vi "Teleop.vi"(10 "Match Info":T2={"Autonomous Elapsed Seconds"=0.0, "TeleOp Elapsed Seconds"=0.0, "Disabled Elapsed Seconds"=0.0, "Visited Autonomous"=FALSE, "Visited TeleOp"=FALSE, "Visited Disabled"=FALSE, "Autonomous Settings"={"Autonomous Style"=enum."Independent", "VI Refnum"=refnum}}, 11 "Call Context":T3) -> ()   [LabVIEW 2012]
doc: "This VI is called for each TeleOp packet received from the DS where the robot is not disabled. It is often used to read from the joysticks and update I/O or to update setpoints for timed control loops. It should complete and return within 20 milliseconds or it may miss DS packets."
uses:
  <vilib>/Rock Robotics/WPI/DriverStation/WPI_DriverStationDerivedRobotMode.ctl
  <vilib>/Rock Robotics/WPI/DriverStation/WPI_DriverStationMatch Info.ctl
  <vilib>/Rock Robotics/WPI/Relay/WPI_RelayValue.ctl
  Robot Global Data.vi
  <vilib>/Rock Robotics/WPI/Joystick/WPI_JoystickGetSetRefNum.vi
panel:
  in  "Roller Speed":dbl=0.75
  in  "RelayValue 2":T1
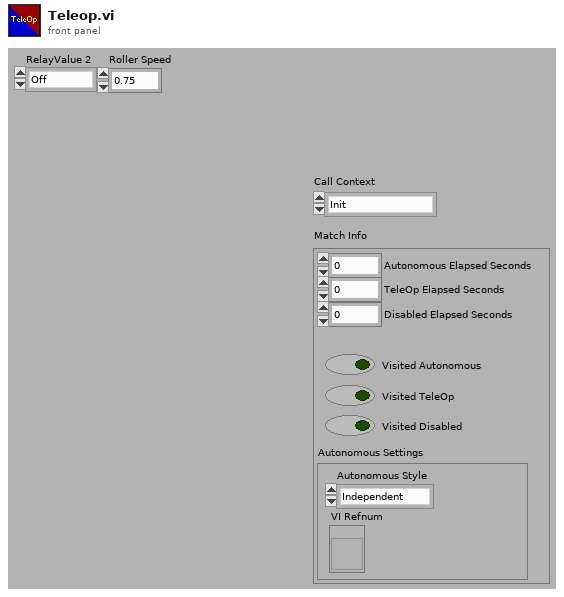
[diagram p1: front panel]
types:
  T1 = typedef "WPI_RelayValue.ctl" = enum16{"Off", "On", "Forward", "Reverse"}
  T2 = typedef "WPI_DriverStationMatch Info.ctl" = cluster{"Autonomous Elapsed Seconds":dbl, "TeleOp Elapsed Seconds":dbl, "Disabled Elapsed Seconds":dbl, "Visited Autonomous":bool, "Visited TeleOp":bool, "Visited Disabled":bool, "Autonomous Settings":cluster{"Autonomous Style":enum16{"Iterative", "Independent"}, "VI Refnum":refnum<vi>}}
  T3 = typedef "WPI_DriverStationDerivedRobotMode.ctl" = enum16{"Init", "Execute", "Stop"}
  T4 = typedef "WPI_ServoDeviceRef.ctl" = cluster{"DeviceStatus":errorcluster, "Digital Module":T5, "PWM Channel":T6, "DeadBand":T7}
  T5 = typedef "FPGA_TypedefDigitalModule.ctl" = enum16{"Digital Module 1", "Digital Module 2"}
  T6 = typedef "FPGA_DIOPWMChannel.ctl" = enum8{"PWM 1", "PWM 2", "PWM 3", "PWM 4", "PWM 5", "PWM 6", "PWM 7", "PWM 8", "PWM 9", "PWM 10", "Invalid"}
  T7 = typedef "WPI_PWMDeadband.ctl" = cluster{"Name":string, "maxPositivePwm":i32, "minPositivePwm":i32, "centerPwm":i32, "maxNegativePwm":i32, "minNegativePwm":i32, "angularRange":u16}
  T8 = typedef "WPI_MotorControlDeviceRef.ctl" = cluster{"DeviceStatus":errorcluster, "Type":enum16{"PWM", "CAN"}, "PWM":cluster{"Digital Module":T5, "PWM Channel":T6, "DeadBand":T7}, "CAN":cluster{"Device Number":u8, "Control Mode":T9, "Semaphore":T10, "Max Vout":dbl}, "Invert":bool, "TransformRef":T11, "InvTransformRef":T11}
  T9 = typedef "WPI_CANJaguar_ControlMode.ctl" = enum8{"Percent VBus", "Current", "Speed", "Position", "Voltage"}
  T10 = typedef "Semaphore RefNum" = refnum<k1>
  T11 = typedef "WPI_PWMTransform_ConPane.ctl" = refnum<vi>
  T12 = typedef "WPI_RelayDevRef.ctl" = cluster{"DevStatus":errorcluster, "Relay Channel":T13, "Digital Module":T5, "Relay Direction":T14}
  T13 = typedef "FPGA_DIORelayChannel.ctl" = enum8{"Relay 1", "Relay 2", "Relay 3", "Relay 4", "Relay 5", "Relay 6", "Relay 7", "Relay 8", "Invalid"}
  T14 = typedef "WPI_RelayDirection.ctl" = enum16{"Both directions", "Forward only", "Reverse only"}
  T15 = cluster{"Driver Station Digital Input (1-8)[0]":bool, "Driver Station Digital Input (1-8)[1]":bool, "Driver Station Digital Input (1-8)[2]":bool, "Driver Station Digital Input (1-8)[3]":bool, "Driver Station Digital Input (1-8)[4]":bool, "Driver Station Digital Input (1-8)[5]":bool, "Driver Station Digital Input (1-8)[6]":bool, "Driver Station Digital Input (1-8)[7]":bool, "Driver Station Digital Input (1-8)[8]":bool}
  T16 = cluster{"Right Servo High":dbl, "Right Servo Mid":dbl, "Right Servo Low":dbl, "Left Servo High":dbl, "Left Servo Mid":dbl, "Left Servo Low":dbl}
  T17 = typedef "WPI_JoystickDevRef.ctl" = cluster{"Device":T18}
  T18 = typedef "WPI_JoystickDeviceEnum.ctl" = enum16{"USB 1", "USB 2", "USB 3", "USB 4", "Kinect 1", "Kinect 2"}
  T19 = cluster{"axis 1 (x)":dbl, "axis 2 (y)":dbl, "axis 3 (throttle)":dbl, "axis 4":dbl, "axis 5":dbl, "axis 6":dbl}
  T20 = typedef "WPI_JoystickButtonState.ctl" = cluster{"Button 1":bool, "Button 2":bool, "Button 3":bool, "Button 4":bool, "Button 5":bool, "Button 6":bool, "Button 7":bool, "Button 8":bool, "Button 9":bool, "Button 10":bool, "Button 11":bool, "Button 12":bool}
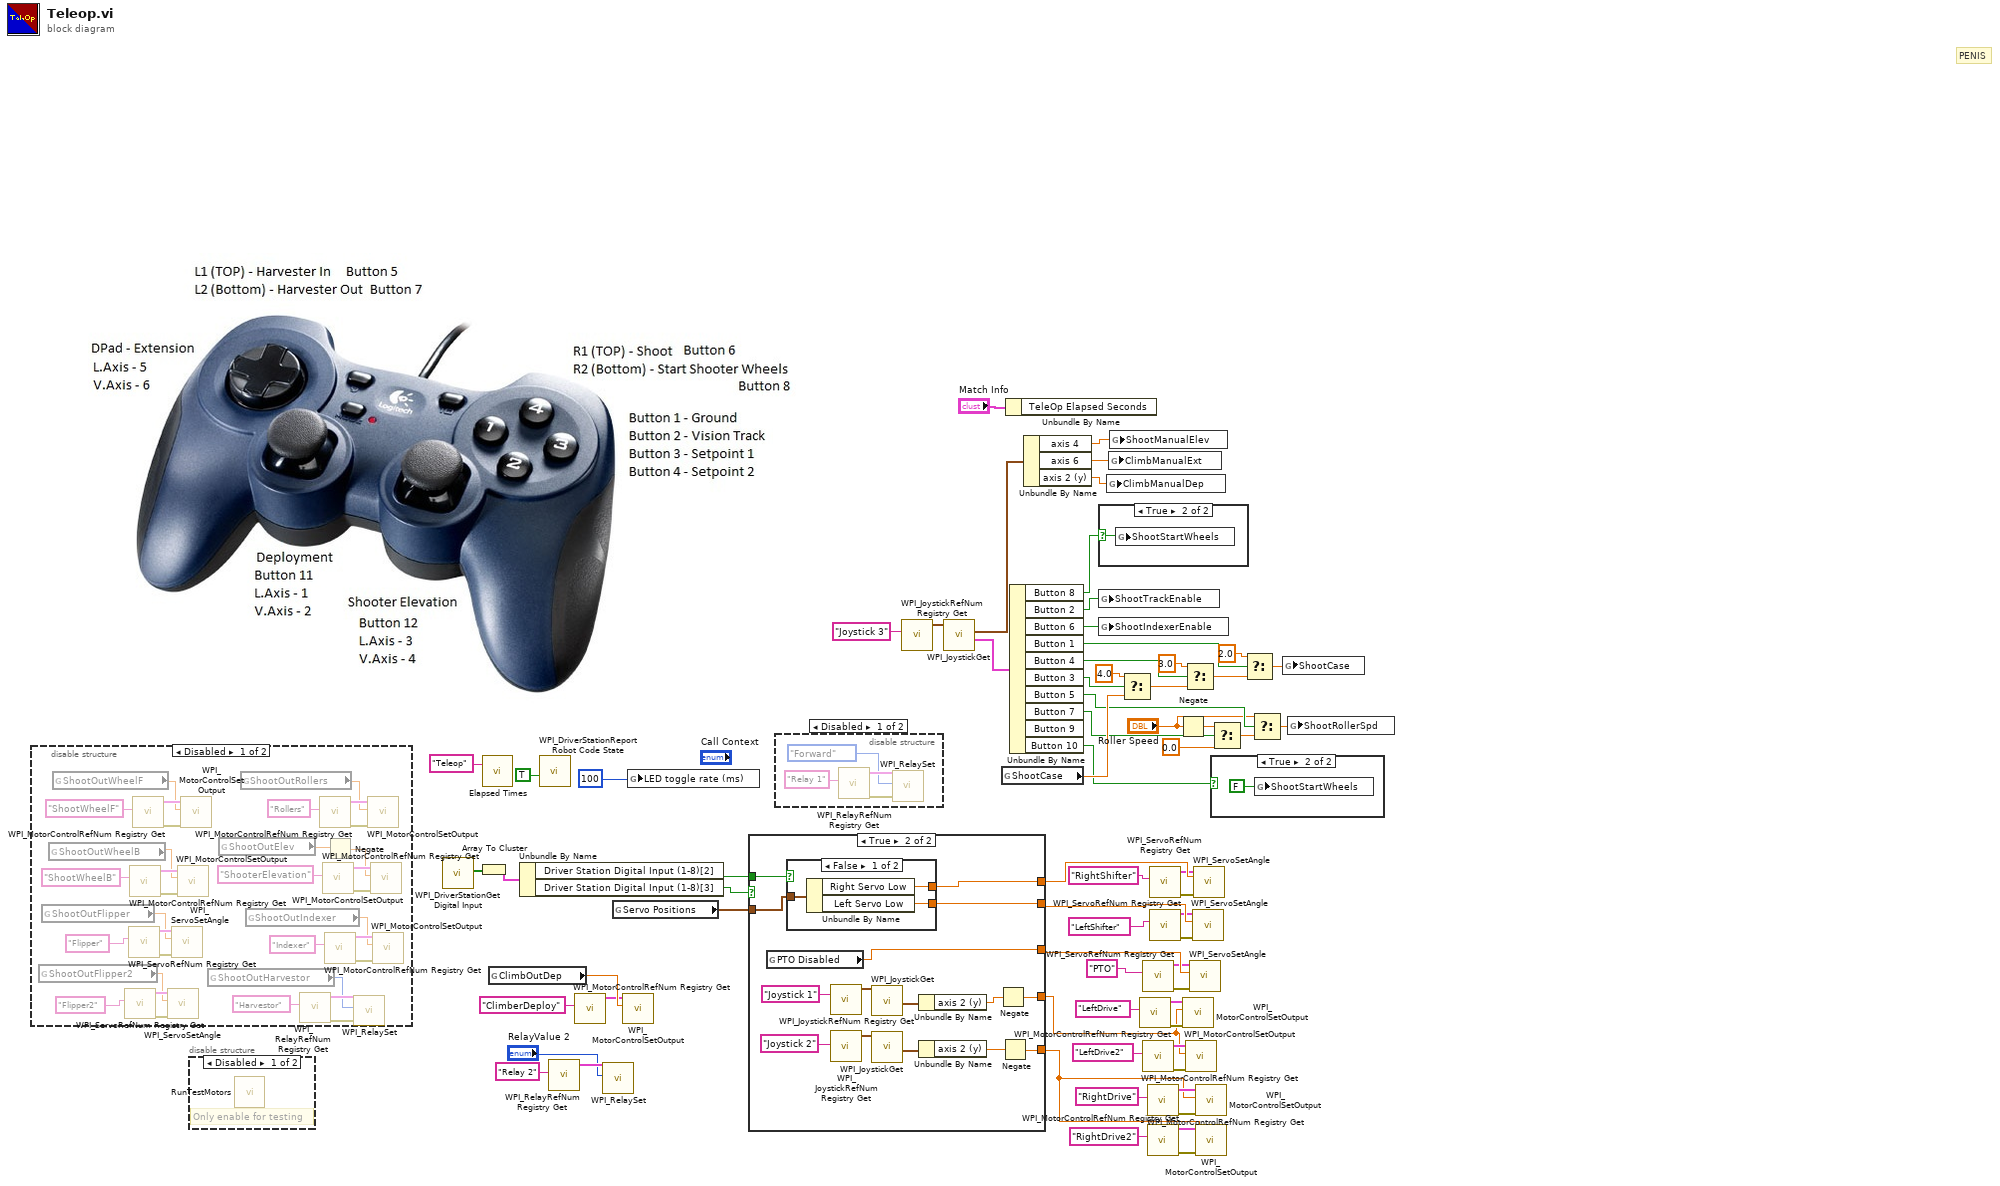
[diagram p0: block diagram]
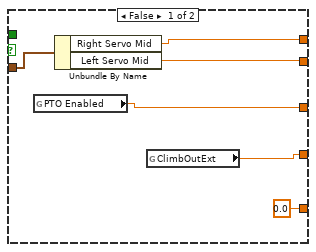
[diagram p2: hidden frame]
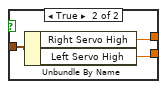
[diagram p3: hidden frame]
diagram:
  # "PENIS"
  n1 = disable-structure shown="Disabled" {
    frame Disabled {
      n2 = global read "Robot Global Data.vi" "ShootOutFlipper2"() -> (w74:dbl)
      n3 = global read "Robot Global Data.vi" "ShootOutFlipper"() -> (w75:dbl)
      n4 = global read "Robot Global Data.vi" "ShootOutWheelB"() -> (w82:dbl)
      n5 = global read "Robot Global Data.vi" "ShootOutWheelF"() -> (w87:dbl)
      n6 = call <vilib>:"WPI_ServoRefNum Registry Get.vi"("refnum name"="Flipper2") -> ("error out"=w78:errorcluster, "ServoDeviceRef"=w77:T4)  [unwired: 9 in]
      n7 = call <vilib>:"WPI_ServoRefNum Registry Get.vi"("refnum name"="Flipper") -> ("error out"=w79:errorcluster, "ServoDeviceRef"=w80:T4)  [unwired: 9 in]
      n8 = call <vilib>:"WPI_MotorControlRefNum Registry Get.vi"("refnum name"="ShootWheelB") -> ("error out"=w97:errorcluster, "MotorControlDevRef"=w98:T8)  [unwired: 9 in]
      n9 = call <vilib>:"WPI_MotorControlRefNum Registry Get.vi"("refnum name"="ShootWheelF") -> ("error out"=w102:errorcluster, "MotorControlDevRef"=w101:T8)  [unwired: 9 in]
      n10 = call <vilib>:"WPI_ServoSetAngle.vi"("error in (no error)"=w78, "Angle"=w74, "ServoDeviceRef"=w77) -> ()  [unwired: 7 in, 2 out]
      n11 = call <vilib>:"WPI_ServoSetAngle.vi"("error in (no error)"=w79, "Angle"=w75, "ServoDeviceRef"=w80) -> ()  [unwired: 7 in, 2 out]
      n12 = call <vilib>:"WPI_MotorControlSetOutput.vi"("error in (no error)"=w97, "Output"=w82, "MotorControlDevRef"=w98) -> ()  [unwired: 6 in, 3 out]
      n13 = call <vilib>:"WPI_MotorControlSetOutput.vi"("error in (no error)"=w102, "Output"=w87, "MotorControlDevRef"=w101) -> ()  [unwired: 6 in, 3 out]
      n14 = global read "Robot Global Data.vi" "ShootOutHarvestor"() -> (w70:T1)
      n15 = global read "Robot Global Data.vi" "ShootOutElev"() -> (w84:dbl)
      n16 = global read "Robot Global Data.vi" "ShootOutRollers"() -> (w85:dbl)
      n17 = global read "Robot Global Data.vi" "ShootOutIndexer"() -> (w86:dbl)
      n18 = call <vilib>:"WPI_RelayRefNum Registry Get.vi"("refnum name"="Harvestor") -> ("error out"=w73:errorcluster, "RelayDevRef"=w71:T12)  [unwired: 9 in]
      n19 = call <vilib>:"WPI_MotorControlRefNum Registry Get.vi"("refnum name"="Rollers") -> ("error out"=w94:errorcluster, "MotorControlDevRef"=w95:T8)  [unwired: 9 in]
      n20 = call <vilib>:"WPI_MotorControlRefNum Registry Get.vi"("refnum name"="ShooterElevation") -> ("error out"=w93:errorcluster, "MotorControlDevRef"=w92:T8)  [unwired: 9 in]
      n21 = Negate(x=w84) -> (-x=w83:dbl)
      n22 = call <vilib>:"WPI_MotorControlRefNum Registry Get.vi"("refnum name"="Indexer") -> ("error out"=w88:errorcluster, "MotorControlDevRef"=w89:T8)  [unwired: 9 in]
      n23 = call <vilib>:"WPI_RelaySet.vi"("error in (no error)"=w73, "RelayValue"=w70, "RelayDevRef"=w71) -> ()  [unwired: 7 in, 2 out]
      n24 = call <vilib>:"WPI_MotorControlSetOutput.vi"("error in (no error)"=w94, "Output"=w85, "MotorControlDevRef"=w95) -> ()  [unwired: 6 in, 3 out]
      n25 = call <vilib>:"WPI_MotorControlSetOutput.vi"("error in (no error)"=w93, "Output"=w83, "MotorControlDevRef"=w92) -> ()  [unwired: 6 in, 3 out]
      n26 = call <vilib>:"WPI_MotorControlSetOutput.vi"("error in (no error)"=w88, "Output"=w86, "MotorControlDevRef"=w89) -> ()  [unwired: 6 in, 3 out]
    }
    frame Enabled {
    }
  }
  n27 = disable-structure shown="Disabled" {
    frame Disabled {
      # "Only enable for testing"
      n28 = call "RunTestMotors.vi"() -> ()  [unwired: 16 in]
    }
    frame Enabled {
    }
  }
  n29 = call <vilib>:"WPI_DriverStationGet Digital Input.vi"() -> ("Driver Station Digital Input (1-8)"=w27:bool[])  [unwired: 11 in]
  n30 = Array To Cluster(array=w27) -> (cluster=w26:T15)
  n31 = call "Elapsed Times.vi"("Call Name"="Teleop") -> ()  [unwired: 2 in, 1 out]
  n32 = global read "Robot Global Data.vi" "ClimbOutDep"() -> (w11:dbl)
  n33 = Unbundle By Name(w26) -> ("Driver Station Digital Input (1-8)[2]"=w25:bool, "Driver Station Digital Input (1-8)[3]"=w17:bool)
  n34 = call <vilib>:"WPI_DriverStationReport Robot Code State.vi"("TeleOp"=TRUE ("Autonomous")) -> ()  [unwired: 10 in, 1 out]
  n35 = call <vilib>:"WPI_RelayRefNum Registry Get.vi"("refnum name"="Relay 2") -> ("RelayDevRef"=w4:T12)  [unwired: 9 in, 1 out]
  n36 = call <vilib>:"WPI_MotorControlRefNum Registry Get.vi"("refnum name"="ClimberDeploy") -> ("MotorControlDevRef"=w9:T8)  [unwired: 9 in, 1 out]
  n37 = call <vilib>:"WPI_RelaySet.vi"("RelayValue"="RelayValue 2", "RelayDevRef"=w4) -> ()  [unwired: 8 in, 2 out]
  n38 = global read "Robot Global Data.vi" "Servo Positions"() -> (w24:T16)
  n39 = call <vilib>:"WPI_MotorControlSetOutput.vi"("Output"=w11, "MotorControlDevRef"=w9) -> ()  [unwired: 7 in, 3 out]
  n40 = global write "Robot Global Data.vi" "LED toggle rate (ms)"(u32 100 ("LED ms toggle rate")) -> ()
  n41 = case shown="True" w17 {
    tunnel: w25 -> [_ w123]
    tunnel: w24 -> [w108 w122]
    tunnel: [w107 w121] -> w23
    tunnel: [w106 w120] -> w22
    tunnel: [w105 w119] -> w14
    tunnel: [w103 w110] -> w13
    tunnel: [0.0 w109] -> w12
    frame False {
      n42 = global read "Robot Global Data.vi" "PTO Enabled"() -> (w105:dbl)
      n43 = Unbundle By Name(w108) -> ("Right Servo Mid"=w107:dbl, "Left Servo Mid"=w106:dbl)
      n44 = global read "Robot Global Data.vi" "ClimbOutExt"() -> (w103:dbl)
    }
    frame True {
      n45 = global read "Robot Global Data.vi" "PTO Disabled"() -> (w119:dbl)
      n46 = case shown="False" w123 {
        tunnel: w122 -> [w126 w129]
        tunnel: [w125 w128] -> w121
        tunnel: [w124 w127] -> w120
        frame False {
          n47 = Unbundle By Name(w126) -> ("Right Servo Low"=w125:dbl, "Left Servo Low"=w124:dbl)
        }
        frame True {
          n48 = Unbundle By Name(w129) -> ("Right Servo High"=w128:dbl, "Left Servo High"=w127:dbl)
        }
      }
      n49 = call <vilib>:"WPI_JoystickRefNum Registry Get.vi"("refnum name"="Joystick 1") -> ("JoystickDevRef"=w111:T17)  [unwired: 1 in, 9 out]
      n50 = call <vilib>:"WPI_JoystickRefNum Registry Get.vi"("refnum name"="Joystick 2") -> ("JoystickDevRef"=w117:T17)  [unwired: 1 in, 9 out]
      n51 = call <vilib>:"WPI_JoystickGet.vi"("JoystickDevRef"=w111) -> ("Axes"=w114:T19)  [unwired: 1 in, 5 out]
      n52 = call <vilib>:"WPI_JoystickGet.vi"("JoystickDevRef"=w117) -> ("Axes"=w118:T19)  [unwired: 1 in, 5 out]
      n53 = Unbundle By Name(w114) -> ("axis 2 (y)"=w113:dbl)
      n54 = Unbundle By Name(w118) -> ("axis 2 (y)"=w115:dbl)
      n55 = Negate(x=w113) -> (-x=w110:dbl)
      n56 = Negate(x=w115) -> (-x=w109:dbl)
    }
  }
  n57 = disable-structure shown="Disabled" {
    frame Disabled {
      n58 = call <vilib>:"WPI_RelayRefNum Registry Get.vi"("refnum name"="Relay 1") -> ("error out"=w131:errorcluster, "RelayDevRef"=w133:T12)  [unwired: 9 in]
      n59 = call <vilib>:"WPI_RelaySet.vi"("error in (no error)"=w131, "RelayValue"=WPI_RelayValue."Forward", "RelayDevRef"=w133) -> ()  [unwired: 7 in, 2 out]
    }
    frame Enabled {
    }
  }
  n60 = call <vilib>:"WPI_JoystickRefNum Registry Get.vi"("refnum name"="Joystick 3") -> ("JoystickDevRef"=w66:T17)  [unwired: 9 in, 1 out]
  n61 = call <vilib>:"WPI_JoystickGet.vi"("JoystickDevRef"=w66) -> ("Buttons"=w64:T20, "Axes"=w63:T19)  [unwired: 4 in, 1 out]
  n62 = global read "Robot Global Data.vi" "ShootCase"() -> (w50:dbl)
  n63 = Unbundle By Name("Match Info") -> ()  [unwired: 1 out]
  n64 = Unbundle By Name(w64) -> ("Button 8"=w43:bool, "Button 2"=w61:bool, "Button 6"=w62:bool, "Button 1"=w58:bool, "Button 4"=w56:bool, "Button 3"=w55:bool, "Button 5"=w46:bool, "Button 7"=w48:bool, "Button 10"=w42:bool)  [unwired: 1 out]
  n65 = Unbundle By Name(w63) -> ("axis 4"=w60:dbl, "axis 6"=w59:dbl, "axis 2 (y)"=w41:dbl)
  n66 = case shown="True" w43 {
    selector: w43 -> [_ w134]
    frame False {
    }
    frame True {
      n67 = global write "Robot Global Data.vi" "ShootStartWheels"(w134) -> ()
    }
  }
  n68 = global write "Robot Global Data.vi" "ShootTrackEnable"(w61) -> ()
  n69 = global write "Robot Global Data.vi" "ShootIndexerEnable"(w62) -> ()
  n70 = global write "Robot Global Data.vi" "ClimbManualDep"(w41) -> ()
  n71 = global write "Robot Global Data.vi" "ClimbManualExt"(w59) -> ()
  n72 = global write "Robot Global Data.vi" "ShootManualElev"(w60) -> ()
  n73 = Select(t=4.0, s=w55, f=w50) -> (s? t:f=w54:dbl)
  n74 = call <vilib>:"WPI_MotorControlRefNum Registry Get.vi"("refnum name"="LeftDrive") -> ("error out"=w32:errorcluster, "MotorControlDevRef"=w35:T8)  [unwired: 9 in]
  n75 = call <vilib>:"WPI_ServoRefNum Registry Get.vi"("refnum name"="PTO") -> ("error out"=w7:errorcluster, "ServoDeviceRef"=w8:T4)  [unwired: 9 in]
  n76 = call <vilib>:"WPI_MotorControlRefNum Registry Get.vi"("refnum name"="LeftDrive2") -> ("error out"=w31:errorcluster, "MotorControlDevRef"=w33:T8)  [unwired: 9 in]
  n77 = call <vilib>:"WPI_MotorControlRefNum Registry Get.vi"("refnum name"="RightDrive") -> ("error out"=w37:errorcluster, "MotorControlDevRef"=w39:T8)  [unwired: 9 in]
  n78 = call <vilib>:"WPI_MotorControlRefNum Registry Get.vi"("refnum name"="RightDrive2") -> ("error out"=w30:errorcluster, "MotorControlDevRef"=w28:T8)  [unwired: 9 in]
  n79 = call <vilib>:"WPI_ServoRefNum Registry Get.vi"("refnum name"="RightShifter") -> ("error out"=w18:errorcluster, "ServoDeviceRef"=w19:T4)  [unwired: 9 in]
  n80 = call <vilib>:"WPI_ServoRefNum Registry Get.vi"("refnum name"="LeftShifter") -> ("error out"=w20:errorcluster, "ServoDeviceRef"=w21:T4)  [unwired: 9 in]
  n81 = Negate(x="Roller Speed") -> (-x=w2:dbl)
  n82 = call <vilib>:"WPI_MotorControlSetOutput.vi"("error in (no error)"=w32, "Output"=w13, "MotorControlDevRef"=w35) -> ()  [unwired: 6 in, 3 out]
  n83 = Select(t=3.0, s=w56, f=w54) -> (s? t:f=w52:dbl)
  n84 = call <vilib>:"WPI_MotorControlSetOutput.vi"("error in (no error)"=w31, "Output"=w13, "MotorControlDevRef"=w33) -> ()  [unwired: 6 in, 3 out]
  n85 = call <vilib>:"WPI_ServoSetAngle.vi"("error in (no error)"=w7, "Angle"=w14, "ServoDeviceRef"=w8) -> ()  [unwired: 7 in, 2 out]
  n86 = call <vilib>:"WPI_ServoSetAngle.vi"("error in (no error)"=w20, "Angle"=w22, "ServoDeviceRef"=w21) -> ()  [unwired: 7 in, 2 out]
  n87 = call <vilib>:"WPI_ServoSetAngle.vi"("error in (no error)"=w18, "Angle"=w23, "ServoDeviceRef"=w19) -> ()  [unwired: 7 in, 2 out]
  n88 = call <vilib>:"WPI_MotorControlSetOutput.vi"("error in (no error)"=w37, "Output"=w12, "MotorControlDevRef"=w39) -> ()  [unwired: 6 in, 3 out]
  n89 = call <vilib>:"WPI_MotorControlSetOutput.vi"("error in (no error)"=w30, "Output"=w12, "MotorControlDevRef"=w28) -> ()  [unwired: 6 in, 3 out]
  n90 = case shown="True" w42 {
    frame False {
    }
    frame True {
      n91 = global write "Robot Global Data.vi" "ShootStartWheels"(FALSE ("ShootStartWheels")) -> ()
    }
  }
  n92 = Select(t=w2, s=w48, f=0.0) -> (s? t:f=w47:dbl)
  n93 = Select(t=2.0, s=w58, f=w52) -> (s? t:f=w49:dbl)
  n94 = Select(t="Roller Speed", s=w46, f=w47) -> (s? t:f=w44:dbl)
  n95 = global write "Robot Global Data.vi" "ShootCase"(w49) -> ()
  n96 = global write "Robot Global Data.vi" "ShootRollerSpd"(w44) -> ()
